vi "EventHandler-Double Click in Mouse Down Event.vi"(3 "max click space(0.2s)":dbl=0.2 format="%#_13g") -> (1 "Double Click?":bool)   [LabVIEW 2017]
doc: "Event handler for a Mouse Down event case that returns TRUE when two clicks arrive within max click space(0.2s) of each other."
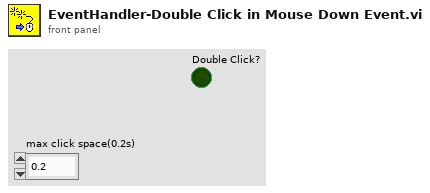
[diagram p1: front panel]
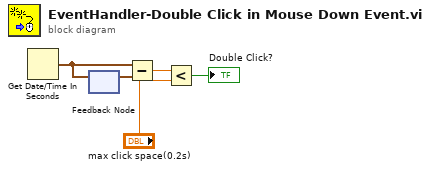
[diagram p0: block diagram]
diagram:
  n1 = Get Date/Time In Seconds() -> (seconds since 1Jan1904=w4:timestamp)
  n2 = feedback #1() -> (w5:timestamp)  [unwired: 1 in]
  n3 = feedback-in #1(w4) -> ()
  n4 = Subtract(x=w4, y=w5) -> (x-y=w3:dbl)
  n5 = Less?(x=w3, y="max click space(0.2s)") -> (x < y?=→"Double Click?":bool)
